vi "Write String Length.vi"(10 "String Length":u32, 11 "RandomStringGenerator in":refnum<class "RandomStringGenerator.lvclass">) -> (3 "RandomStringGenerator out":refnum<class "RandomStringGenerator.lvclass">)   [LabVIEW 2014, in "RandomStringGenerator.lvclass"]
uses:
  RandomStringGenerator.lvclass
  RandomStringGenerator.lvclass/RandomStringGenerator.ctl
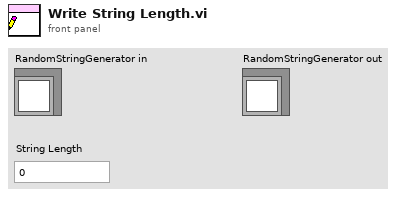
[diagram p1: front panel]
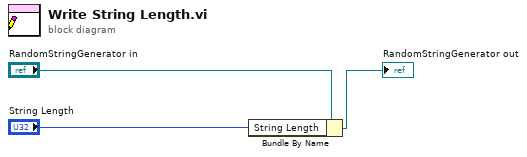
[diagram p0: block diagram]
diagram:
  n1 = Bundle By Name(cluster="RandomStringGenerator in", "String Length"="String Length") -> (→"RandomStringGenerator out":refnum<class "RandomStringGenerator.lvclass">)
